vi "ConvertArmSourceToString.vi"(11 "Arm Source":T1) -> (3 "Arm Source String":string)   [LabVIEW 2012, in "Keithley-7001.lvlib"]
uses:
  Keithley-7001.lvlib
  Public/Controls/ArmSource.ctl
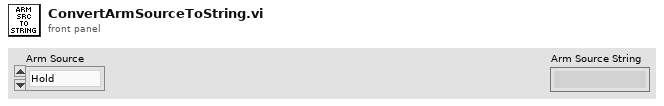
[diagram p1: front panel]
types:
  T1 = typedef "Keithley-7001.lvlib/ArmSource.ctl" = enum16{"Hold", "Immediate", "Manual", "Bus", "TLink", "External"}
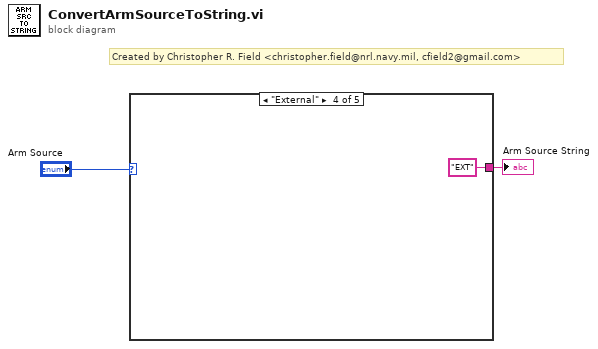
[diagram p0: block diagram]
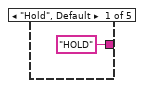
[diagram p2: hidden frame]
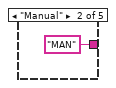
[diagram p3: hidden frame]
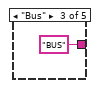
[diagram p4: hidden frame]
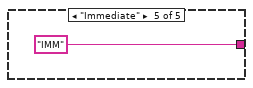
[diagram p5: hidden frame]
diagram:
  # "Created by Christopher R. Field <christopher.field@nrl.navy.mil, cfield2@gmail.com>"
  n1 = case shown="\"External\"" "Arm Source" {
    tunnel: ["HOLD" "MAN" "BUS" "EXT" "IMM"] -> w1
    frame "Hold", Default {
    }
    frame "Manual" {
    }
    frame "Bus" {
    }
    frame "External" {
    }
    frame "Immediate" {
    }
  }
  "Arm Source String" <- w1
